vi "Write Response.vi"(6 "overwrite on timeout (T)":bool, 8 "error in (no error)":errorcluster, 9 "timeout in ms (0)":i32, 10 "response":T1, 11 "Interface in":refnum<class "Engine Interface.lvclass">) -> (0 "error out":errorcluster, 1 "timed out?":bool, 3 "Interface out":refnum<class "Engine Interface.lvclass">)   [LabVIEW 2017, in "Data Sharing Framework Core.lvlib" / "Data Sharing Framework Engine.lvlib" / "Engine Interface.lvclass"]
uses:
  Engine Interface/Engine Interface.lvclass
  Engine Interface/16B Data.ctl
  Engine Interface/16B Payload.ctl
  Engine Interface/Engine Interface.lvclass/Engine Interface.ctl
  Debug/Debug Flags FIFO/Debug Flags FIFO.lvclass/Debug Flags FIFO.ctl
  Debug/Debug Flags FIFO/Get Infinite Timeouts.vi
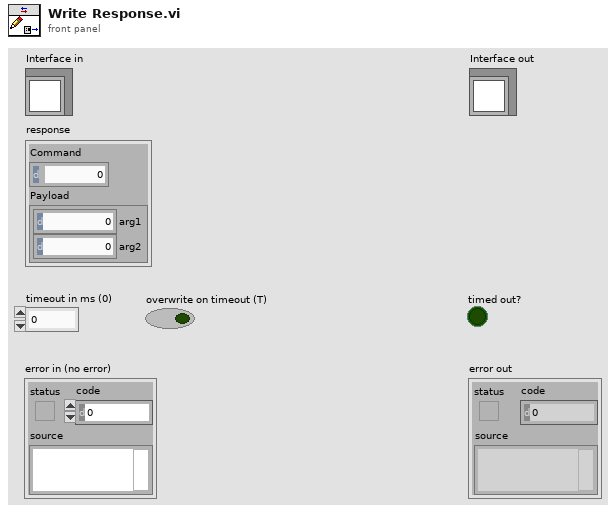
[diagram p1: front panel]
types:
  T1 = typedef "Data Sharing Framework Core.lvlib/Data Sharing Framework Engine.lvlib/Engine Interface.lvclass/16B Data.ctl" = cluster{"Command":u8, "Payload":T2}
  T2 = typedef "Data Sharing Framework Core.lvlib/Data Sharing Framework Engine.lvlib/Engine Interface.lvclass/16B Payload.ctl" = cluster{"arg1":u64, "arg2":u64}
  T3 = typedef "Data Sharing Framework Core.lvlib/Data Sharing Framework Engine.lvlib/Engine Interface.lvclass/16B RT FIFO Reference.ctl" = refnum<k33>
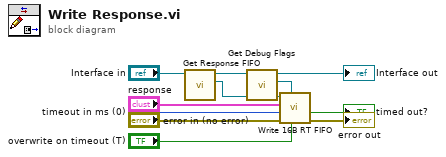
[diagram p0: block diagram]
diagram:
  n1 = call "Get Response FIFO.vi"("Interface in"="Interface in") -> ("Response FIFO"=w11:T3, "Interface out"=w7:refnum<class "Engine Interface.lvclass">)  [unwired: 9 in]
  n2 = call "Get Debug Flags.vi"("Interface in"=w7) -> ("FIFO Debug Flags"=w6:refnum<class "Debug Flags FIFO.lvclass">, "Interface out"=→"Interface out":refnum<class "Engine Interface.lvclass">)  [unwired: 9 in]
  n3 = call "Write 16B RT FIFO.vi"("overwrite on timeout (T)"="overwrite on timeout (T)", "FIFO Debug Flags"=w6, "error in (no error)"="error in (no error)", "timeout in ms (0)"="timeout in ms (0)", "element"="response", "RT FIFO in"=w11) -> ("error out"=→"error out":errorcluster, "timed out?"=→"timed out?":bool)  [unwired: 3 in, 1 out]
